vi "Table Value To 2D I32.vi"(11 "Table Ref In":refnum<vi>) -> (1 "I32 Out":i32[][](array[numeric]), 3 "Table Ref Out":refnum<vi>)   [LabVIEW 2024]
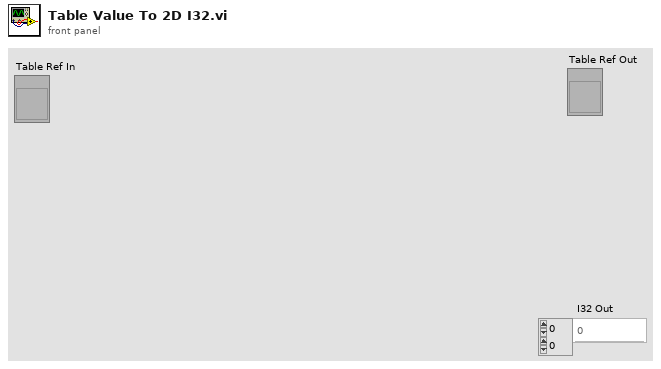
[diagram p1: front panel]
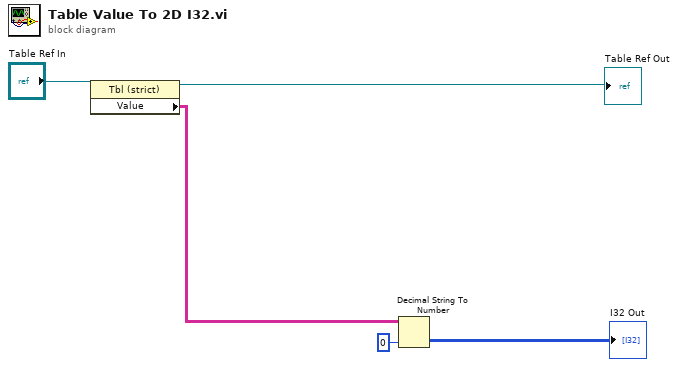
[diagram p0: block diagram]
diagram:
  n1 = property class="Tbl (strict)"(reference="Table Ref In") -> (reference out=→"Table Ref Out":refnum<vi>, "Value"=w3:string[][])  [unwired: 1 in, 1 out]
  n2 = Decimal String To Number(string=w3, default (0L)=0 ("default (0 I32)")) -> (number=→"I32 Out":i32[][])  [unwired: 1 in, 1 out]
